vi "sin graph.vi"() -> ()   [LabVIEW 2021]
panel:
  out "Waveform Chart":dbl(graph)
  in  "Numeric":dbl
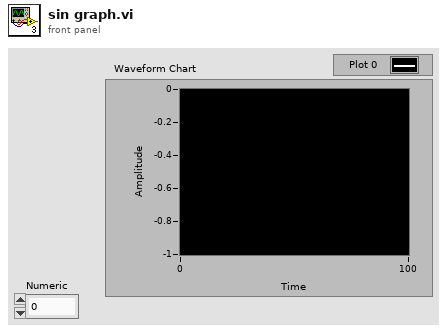
[diagram p1: front panel]
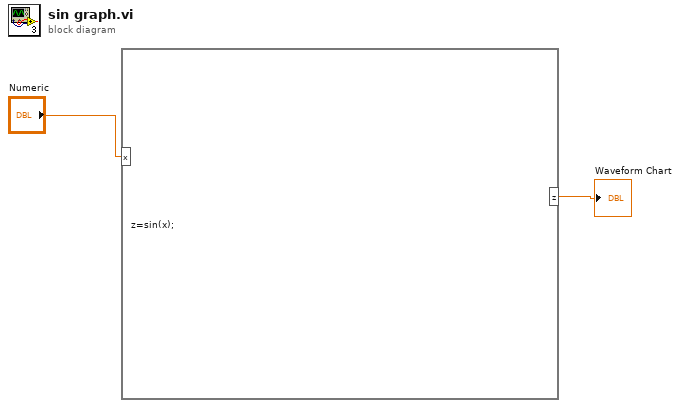
[diagram p0: block diagram]
diagram:
  n1 = formula code="z=sin(x);"("x"="Numeric") -> ("z"=→"Waveform Chart":dbl)
